vi "p4y2.vi"() -> ()   [LabVIEW 2020]
uses:
  <vilib>/Utility/file.llb/Read Delimited Spreadsheet (DBL).vi
  <vilib>/Utility/file.llb/Write Delimited Spreadsheet (string).vi
  <vilib>/gmath/NI_Gmath.lvlib
panel:
  in  "String 2":string="Tiideberg,"
  in  "String":string="Alar,"
  in  "file path (dialog if empty)":path=path "C:/Users/Oliver/Documents/uus.csv"
  out "Waveform Graph":T1(graph)=[{"disabled index (col)"=0, "disabled index (col)"=1, "Array"=[5.7, 5.7, 5.7, 5.7, 5.7, 5.7, 5.7, 5.7, 5.7, 5.7, 5.7, 6.6, 7.6, 9.1, 8.7, 8.0, 8.1, 8.8, 9.4, 10.0, 9.4, 8.4, 6.4, 4.3, 3.8, 3.8, 3.4, 2.5, 1.8, 1.2, 0.9, 1.0, 1.1, 1.3, 1.1, 1.1, 0.8, 0.8, 0.8, 0.9, 0.9, 1.0, 0.9, 0.8, 0.9, 1.6, 2.4, 2.4, 2.5, 2.4, 2.3, 2.2, 2.3, 2.2, 2.5, 1.8, 1.0, 0.8, 0.8, 1.1, 1.3, 1.3, 1.5, 1.6, 1.2, 1.5, 1.9, 2.8, 4.0, 4.5, 5.0, 5.0, 5.8, 7.9, 9.0, 9.5, 10.5, 10.1, 9.4, 9.5, 9.5, 9.4, 8.6, 7.1, 6.6, 5.9, 5.3, 5.5, 6.9, 7.7, 9.1, 9.8, 9.8, 11.0, 12.1, 13.3, 14.3, 15.6, 14.6, 13.1, 13.0, 14.3, 16.6, 16.3, 18.1, 19.2, 19.0, 20.2, 21.4, 22.7, 23.9, 24.2, 23.7, 24.3, 23.2, 24.1, 24.6, 25.0, 28.9, 32.3, 30.8, 32.0, 35.6, 37.8, 39.5, 40.8, 42.2, 45.3, 44.0, 44.7, 51.0, 53.2, 54.4, 52.9, 49.8, 49.3, 48.3, 49.2, 49.3, 47.4, 41.3, 37.4, 32.9, 34.0, 36.3, 35.8, 36.9, 31.9, 27.7, 28.2, 30.8, 36.5, 39.4, 40.6, 43.3, 41.3, 41.4, 51.4, 58.6, 63.9, 72.7, 73.3, 74.2, 77.0, 91.8, 103.2, 123.6, 133.8, 145.2, 148.2, 147.7, 152.8, 184.1, 201.9, 207.5, 216.8, 213.8, 209.6, 217.4, 246.0, 269.1, 286.0, 283.4, 280.8, 274.8, 290.6, 310.9, 328.9, 339.3, 333.7, 323.4, 312.2, 329.7, 351.5, 378.1, 395.9, 402.5, 390.6, 381.7, 400.7, 429.5, 446.5, 470.0, 459.1, 445.2, 418.9, 429.8, 478.4, 515.4, 517.3, 520.9, 513.4, 493.9, 526.2, 562.7, 590.4, 576.0, 539.1, 515.2, 506.4, 544.9, 589.7, 575.0, 546.5, 511.1, 492.8, 491.3, 526.9, 593.7, 624.7, 583.5, 552.7, 539.9, 535.6, 586.8, 610.8, 613.1, 602.8, 533.0, 480.9, 485.4, 503.4, 541.3, 557.3, 520.2, 510.2, 490.7, 464.7, 489.9, 532.4, 541.3, 521.0, 500.9, 488.1, 480.2, 495.9, 537.1, 560.6, 555.4, 528.5, 493.8, 507.9, 541.0, 571.8, 602.6, 609.6, 609.4, 591.7, 594.5, 633.5, 699.0, 740.0, 738.9, 729.6, 741.2, 761.5, 801.3, 875.0, 933.8, 1009.8, 1030.3, 1037.7, 1070.0, 1158.3, 1217.3, 1274.5, 1321.9, 1338.7, 1336.4, 1310.0, 1338.3, 1431.4, 1456.2, 1468.3, 1419.7, 1394.5, 1386.7, 1433.0, 1484.8, 1529.1]}, {"disabled index (col)"=0, "disabled index (col)"=1, "Array"=[0.0025519, 0.0025519, 0.0025519, 0.0025519, 0.0025519, 0.0025519, 0.0025519, 0.0025519, 0.0025519, 0.0025519, 0.0025519, 0.002559100000000001, 0.002566, 0.0025742, 0.0025817, 0.0025872, 0.0025886999999999998, 0.002586, 0.0025868, 0.0025719, 0.0025659999999999997, 0.0025596, 0.0025513000000000003, 0.0025431000000000004, 0.0025317, 0.002521, 0.0025082999999999993, 0.0024963999999999997, 0.0024824, 0.0024802, 0.0024757, 0.0024713, 0.002458, 0.0024488, 0.0024361, 0.0024234, 0.0024117, 0.0023972999999999998, 0.0023837, 0.0023698, 0.0023561, 0.0023399, 0.0023321999999999996, 0.0023208, 0.0023650999999999993, 0.0025329, 0.0027367, 0.0029138000000000002, 0.0030353000000000003, 0.0031839, 0.0033026, 0.0033844000000000005, 0.0034749000000000004, 0.0035520000000000005, 0.0035742000000000005, 0.0035110000000000002, 0.0034302, 0.0033601, 0.0033324, 0.0032749, 0.0032505, 0.0032581, 0.0032621000000000004, 0.0032797, 0.0032984, 0.0032741, 0.0032429, 0.0032218999999999998, 0.003217, 0.0032203999999999996, 0.003255, 0.0032742, 0.0032871999999999997, 0.0033202999999999996, 0.0033472000000000003, 0.0033920000000000005, 0.0034183, 0.0034503, 0.0034795, 0.0035066, 0.003481, 0.0034901000000000003, 0.0034980000000000002, 0.003492, 0.0034984, 0.0034886, 0.0035061000000000003, 0.0035061999999999997, 0.0034974, 0.0034901999999999997, 0.0034909999999999997, 0.0034814, 0.003477, 0.0034657, 0.0034402, 0.0034197000000000003, 0.003374, 0.0033528000000000004, 0.0033447999999999998, 0.0033264, 0.0033119000000000004, 0.0032938000000000004, 0.0032603, 0.0032004000000000004, 0.0031634000000000002, 0.0031068, 0.0030632, 0.0030134000000000003, 0.0029515, 0.002902, 0.002855, 0.0028113, 0.0027834, 0.0027796, 0.0027694, 0.0027777, 0.0027794000000000004, 0.0027826000000000005, 0.002791, 0.0027909, 0.0027937, 0.0027768, 0.0027593, 0.0027418, 0.0027294999999999997, 0.0027184, 0.0027108, 0.0027015, 0.0026914, 0.0026785, 0.0026647, 0.0026646, 0.0026607999999999996, 0.0026615, 0.0026558000000000003, 0.0026475, 0.0026339, 0.0026213000000000005, 0.0026155000000000006, 0.0026183, 0.0026195000000000003, 0.0026262, 0.0026322999999999997, 0.0026364, 0.0026361, 0.0026339, 0.0026347000000000002, 0.0026347000000000002, 0.0026302, 0.0026209, 0.0026168000000000003, 0.0026133999999999997, 0.0026133999999999997, 0.0026124999999999994, 0.0026165999999999997, 0.002644, 0.0026539, 0.0026632, 0.0026661000000000002, 0.0026632, 0.0026568, 0.0026495, 0.002641, 0.0026267, 0.0026124, 0.0025822, 0.0025808000000000003, 0.0025926, 0.0026008, 0.0026159, 0.0026281000000000004, 0.0026521, 0.0026722000000000004, 0.002703, 0.0027275, 0.0027465, 0.0027558999999999995, 0.0027683, 0.0027973, 0.0028171, 0.0028415, 0.0028802, 0.002941, 0.0029934000000000002, 0.0030886000000000004, 0.0032063, 0.0032559999999999998, 0.0032931, 0.0033204000000000003, 0.0033672, 0.0034277, 0.0034543000000000004, 0.0034497, 0.0034567, 0.0034265000000000003, 0.0033657, 0.0033794999999999997, 0.0033866999999999994, 0.0033963999999999995, 0.0033679, 0.0033304, 0.003291, 0.0032742, 0.0032508000000000003, 0.003234, 0.0032223, 0.0032023000000000004, 0.0032088000000000004, 0.0032511000000000007, 0.0033311, 0.0034039, 0.0035842, 0.0037467, 0.0038877999999999994, 0.003948, 0.0040748, 0.0042021, 0.0043186000000000006, 0.0043989, 0.0044528, 0.0045148, 0.0044892000000000005, 0.004500499999999999, 0.0047634999999999995, 0.0054608, 0.0060925, 0.0065622, 0.0071346, 0.007701799999999999, 0.0082065, 0.0087713, 0.009333999999999999, 0.0097415, 0.009883800000000002, 0.0095834, 0.0093413, 0.009361600000000001, 0.009264, 0.0091543, 0.0091022, 0.009009099999999999, 0.008886100000000003, 0.008870800000000002, 0.008833299999999999, 0.0089143, 0.0089422, 0.008885, 0.008780199999999998, 0.0086702, 0.0088475, 0.0089301, 0.0118587, 0.013722799999999999, 0.0168835, 0.019323899999999998, 0.0217196, 0.024802700000000004, 0.028460000000000003, 0.0324169, 0.036689700000000006, 0.0428638, 0.04710569999999999, 0.051332199999999994, 0.054597799999999995, 0.0578104, 0.06149639999999999, 0.0639177, 0.064418, 0.06552109999999998, 0.06540189999999999, 0.0634415, 0.06106170000000002, 0.0595219, 0.05783579999999999, 0.057063699999999995, 0.055192399999999996, 0.0538347, 0.054407300000000006, 0.0536185, 0.05353599999999999, 0.05311790000000001, 0.052313399999999996, 0.052066999999999995, 0.0515687, 0.0508208, 0.050645699999999995, 0.05076519999999999, 0.0503279, 0.050698, 0.05152260000000001, 0.052303699999999995, 0.052995099999999996, 0.0534023, 0.05386339999999999, 0.0550691, 0.0560865, 0.05658529999999999, 0.057287, 0.0576415, 0.05741430000000001]}]
  in  "Aknasuurus KOVIDTSOK":i32=10
  in  "Päevade arv":i32=300
  in  "delimiter (\\t) 2":string=","
  in  "format (%s) 2":string="%s"
  in  "file path (use dialog) 2":path=path "C:/Users/Oliver/Downloads/HistoricalData_1616255744025.csv"
  in  "delimiter (\\t)":string=","
  in  "format (%s)":string="%s"
  in  "file path (use dialog)":path=path "C:/Users/Oliver/Downloads/opendata_covid19_tests_total.csv"
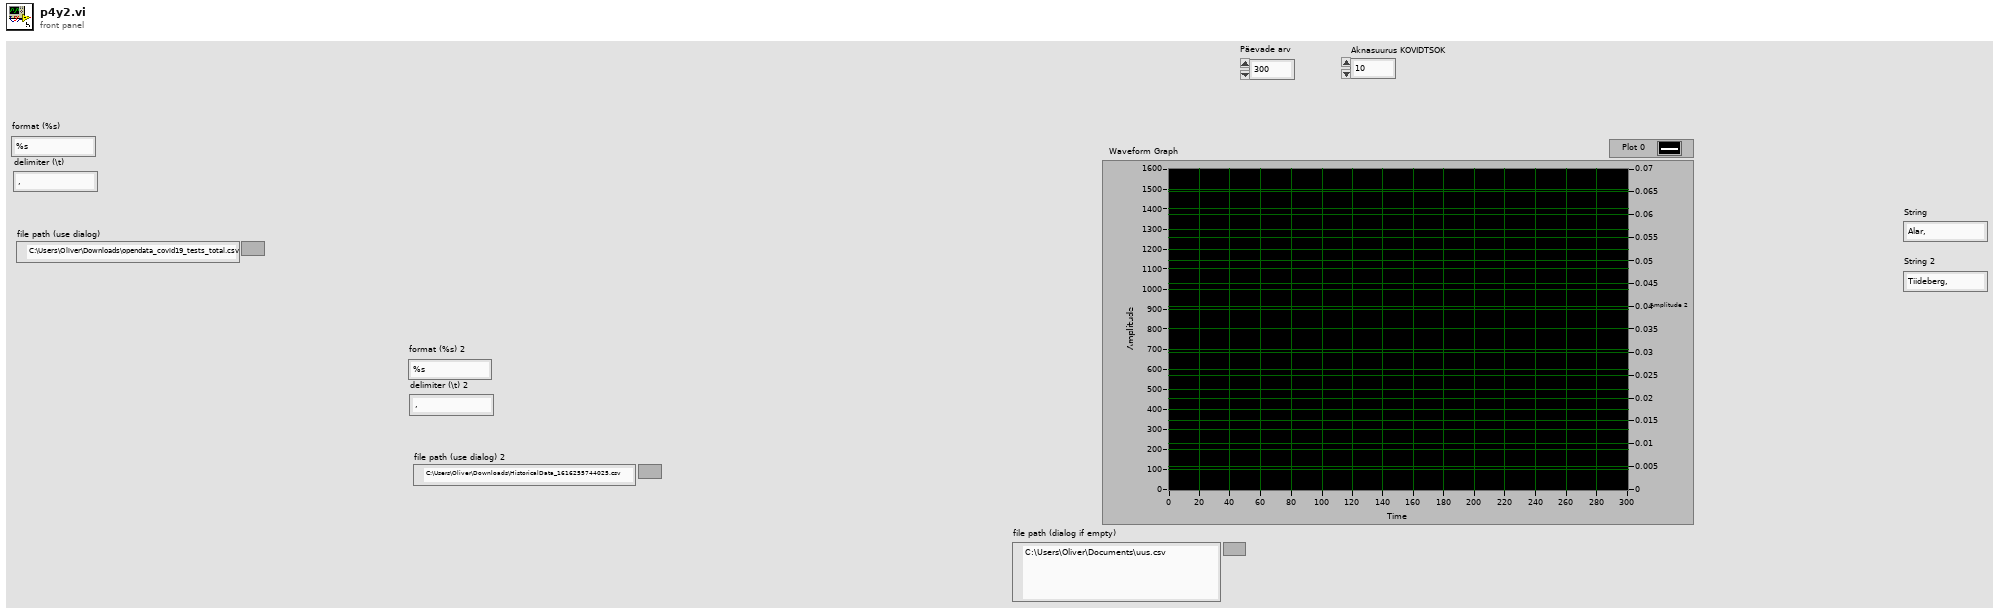
[diagram p1: front panel]
types:
  T1 = cluster{"disabled index (col)":i32, "disabled index (col)":i32, "Array":dbl[]}[]
  T2 = cluster{"disabled index (col)":i32, "disabled index (col)":i32, "Array":dbl[]}
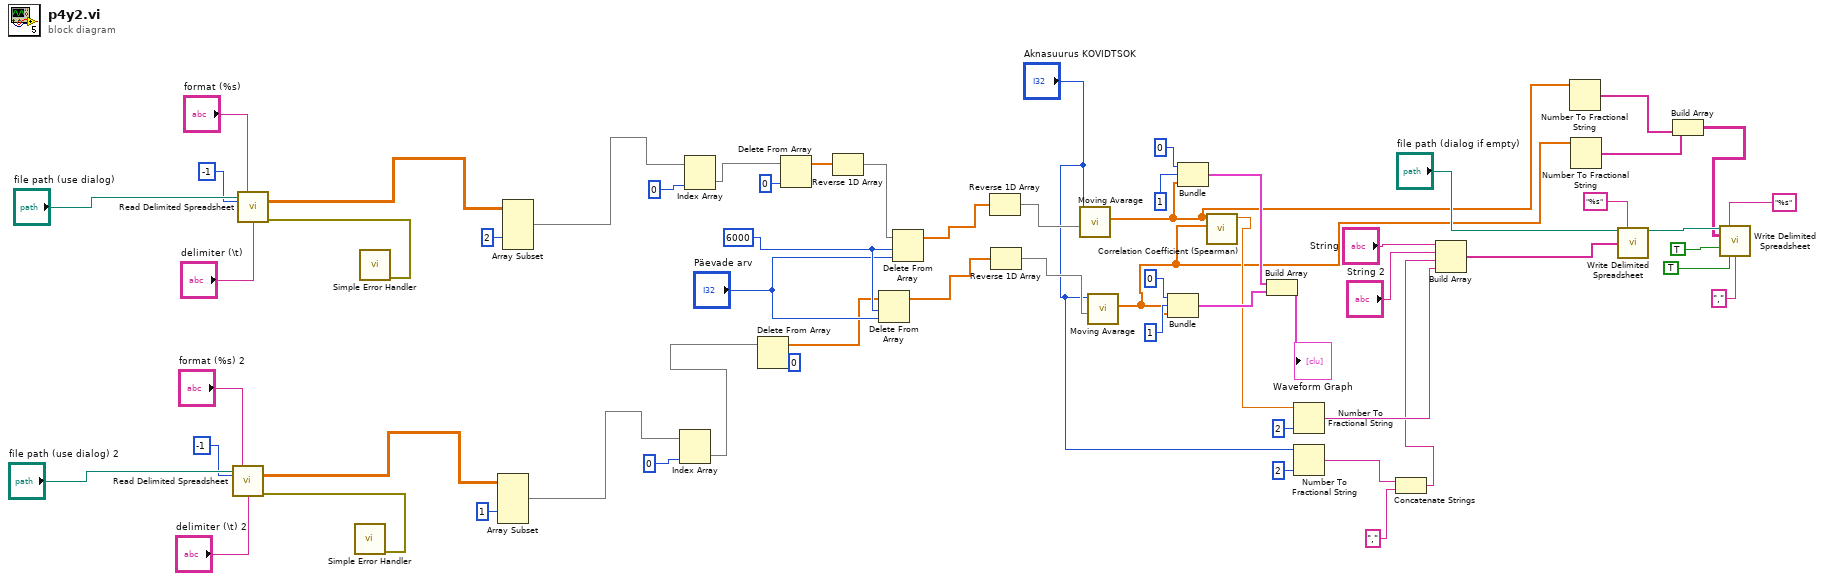
[diagram p0: block diagram]
diagram:
  w37 = 6000 ("index")
  n1 = call-poly <vilib>:"Read Delimited Spreadsheet.vi"("file path (dialog if empty)"="file path (use dialog) 2", "format (%.3f)"="format (%s) 2", "number of rows (all:-1)"=-1, "delimiter (\\t)"="delimiter (\\t) 2") -> ("all rows"=w47:dbl[][], "error out"=w51:errorcluster)  [unwired: 6 in, 4 out]
  n2 = call-poly <vilib>:"Read Delimited Spreadsheet.vi"("file path (dialog if empty)"="file path (use dialog)", "format (%.3f)"="format (%s)", "number of rows (all:-1)"=-1, "delimiter (\\t)"="delimiter (\\t)") -> ("all rows"=w56:dbl[][], "error out"=w60:errorcluster)  [unwired: 6 in, 4 out]
  n3 = call <vilib>:"Simple Error Handler.vi"("error in (no error)"=w51) -> ()  [unwired: 4 in, 5 out]
  n4 = call <vilib>:"Simple Error Handler.vi"("error in (no error)"=w60) -> ()  [unwired: 4 in, 5 out]
  n5 = Array Subset(array=w47, index (col)=1 ("index")) -> (w45:dbl[][])  [unwired: 3 in]
  n6 = Array Subset(array=w56, index (col)=2 ("index")) -> (w54:dbl[][])  [unwired: 3 in]
  n7 = Index Array(array=w45, index (col)=0 ("disabled index (col)")) -> (element=w43:dbl[])  [unwired: 1 in]
  n8 = Index Array(array=w54, index (col)=0 ("disabled index (col)")) -> (element=w40:dbl[])  [unwired: 1 in]
  n9 = Delete From Array(array=w43, index=0) -> (array with subset deleted=w35:dbl[])  [unwired: 1 in, 1 out]
  n10 = Delete From Array(array=w40, index=0) -> (array with subset deleted=w39:dbl[])  [unwired: 1 in, 1 out]
  n11 = Reverse 1D Array(array=w39) -> (reversed array=w38:dbl[])
  n12 = Delete From Array(array=w35, length=w37, index="Päevade arv") -> (array with subset deleted=w25:dbl[])  [unwired: 1 out]
  n13 = Delete From Array(array=w38, length=w37, index="Päevade arv") -> (array with subset deleted=w27:dbl[])  [unwired: 1 out]
  n14 = Reverse 1D Array(array=w27) -> (reversed array=w26:dbl[])
  n15 = Reverse 1D Array(array=w25) -> (reversed array=w24:dbl[])
  n16 = call "Moving Avarage.vi"("array"=w26, "Aknasuurus"="Aknasuurus KOVIDTSOK") -> ("Array"=w7:dbl[])  [unwired: 9 in]
  n17 = call "Moving Avarage.vi"("array"=w24, "Aknasuurus"="Aknasuurus KOVIDTSOK") -> ("Array"=w6:dbl[])  [unwired: 9 in]
  n18 = Bundle("disabled index (col)"=0, "disabled index (col)"=1, "Array"=w6) -> (w31:T2)  [unwired: 1 in]
  n19 = Bundle("disabled index (col)"=0, "disabled index (col)"=1, "Array"=w7) -> (w28:T2)  [unwired: 1 in]
  n20 = call <vilib>:"Correlation Coefficient (Spearman).vi"("Y"=w6, "X"=w7) -> ("correlation coefficient r"=w21:dbl)  [unwired: 8 in, 1 out]
  n21 = Build Array(w28, w31) -> (→"Waveform Graph":T1)
  n22 = Number To Fractional String(number=w21, precision (6)=i16 2) -> (F-format string=w13:string)  [unwired: 2 in]
  n23 = Number To Fractional String(number="Aknasuurus KOVIDTSOK", precision (6)=i16 2) -> (F-format string=w11:string)  [unwired: 2 in]
  n24 = Concatenate Strings(w11, "," ("string")) -> (w10:string)
  n25 = Build Array("String", "String 2", w10, w13) -> (w16:string[])
  n26 = Number To Fractional String(number=w7) -> (F-format string=w2:string[])  [unwired: 3 in]
  n27 = Number To Fractional String(number=w6) -> (F-format string=w3:string[])  [unwired: 3 in]
  n28 = call-poly <vilib>:"Write Delimited Spreadsheet.vi"("file path (dialog if empty)"="file path (dialog if empty)", "format (%s)"="%s", "1D data"=w16) -> ("new file path (Not A Path if cancelled)"=w18:path)  [unwired: 11 in, 1 out]
  n29 = Build Array(w3, w2) -> (w1:string[][])
  n30 = call-poly <vilib>:"Write Delimited Spreadsheet.vi"("file path (dialog if empty)"=w18, "format (%s)"="%s" ("format (%.3f)"), "2D data"=w1, "append to file? (new file:F)"=TRUE, "transpose? (no:F)"=TRUE, "delimiter (\\t)"="," ("delimiter (\\t)")) -> ()  [unwired: 8 in, 2 out]
